vi "Oscilloscope Measure.vi"(8 "error in (no error)":errorcluster, 11 "Oscilloscope in":refnum<class "Oscilloscope.lvclass">) -> (0 "error out":errorcluster, 3 "Oscilloscope out":refnum<class "Oscilloscope.lvclass">)   [LabVIEW 2023, in "HardwareAbstractionLayer_LVOOP.lvlib" / "Oscilloscope.lvclass"]
uses:
  Oscilloscope.lvclass
panel:
  out "instrument handle out":refnum<k15>
  in  "instrument handle":refnum<k15>
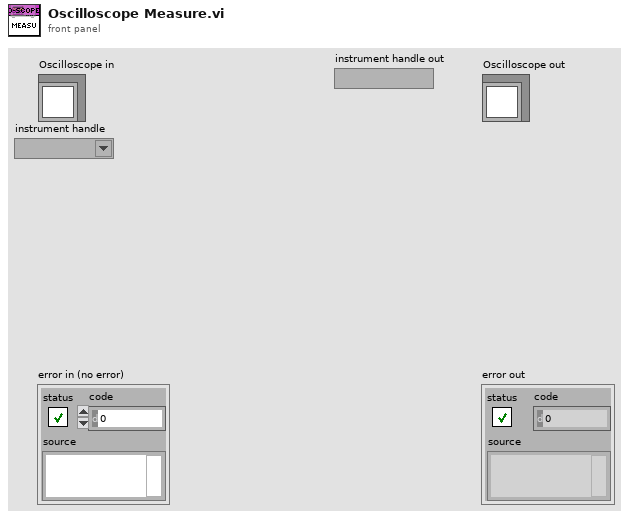
[diagram p1: front panel]
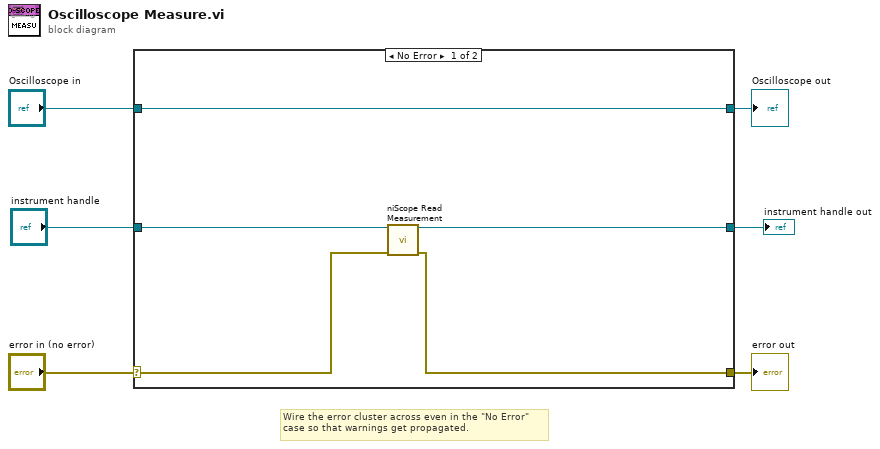
[diagram p0: block diagram]
diagram:
  # "Wire the error cluster across even in the \"No Error\"\ncase so that warnings get propagated."
  n1 = case shown="No Error" "error in (no error)" {
    selector: "error in (no error)" -> [w9 w14]
    tunnel: [w8 w14] -> w5
    tunnel: [w11 w13] -> w3
    tunnel: "Oscilloscope in" -> [w11 w13]
    tunnel: "instrument handle" -> [w10 w12]
    tunnel: [w7 w12] -> w1
    frame No Error {
      n2 = call <instrlib>:"niScope Read Measurement.vi"("instrument handle"=w10, "error in"=w9) -> ("instrument handle out"=w7:refnum<k15>, "error out"=w8:errorcluster)  [unwired: 11 in, 1 out]
    }
    frame Error {
    }
  }
  "error out" <- w5
  "Oscilloscope out" <- w3
  "instrument handle out" <- w1
